vi "OpenNetworkStreamWriter.vi"(6 "E-Stop DVR":refnum<data-value>, 8 "error in (no error)":errorcluster, 11 "Writer Parameters":T1) -> (0 "error out":errorcluster, 2 "Time Opened":timestamp, 3 "Writer Endpoint":refnum<k21>, 4 "Aborted?":bool)   [LabVIEW 2012, in "NetworkStreamWriter.lvclass"]
doc: "Opens a network stream writer endpoint. This VI persistently tries to open the connection until it is successful or the e-stop is triggered by-reference (data value reference). The e-stop will be triggered by the Close method of the owning Object.\n\nJared Kirschner, 2012."
uses:
  NetworkStreamWriter.lvclass
  WriterParameters.ctl
  Shared/ElapsedTimeMessage.ctl
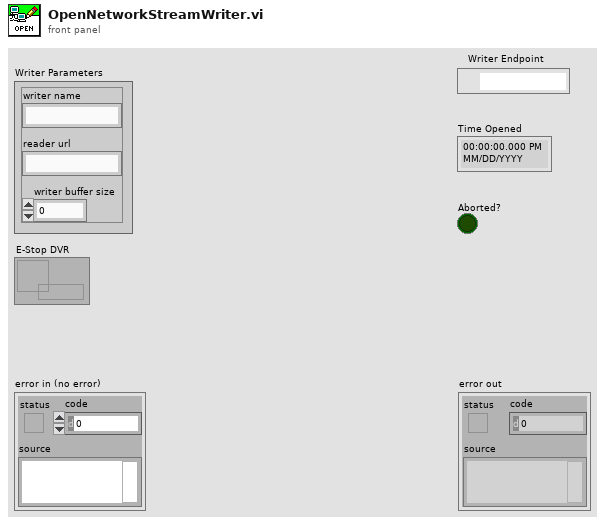
[diagram p1: front panel]
types:
  T1 = typedef "NetworkStreamWriter.lvclass/WriterParameters.ctl" = cluster{"writer name":string, "reader url":string, "writer buffer size":i32}
  T2 = typedef "ElapsedTimeMessage.ctl" = cluster{"Data":variant, "Elapsed Time (s)":dbl}
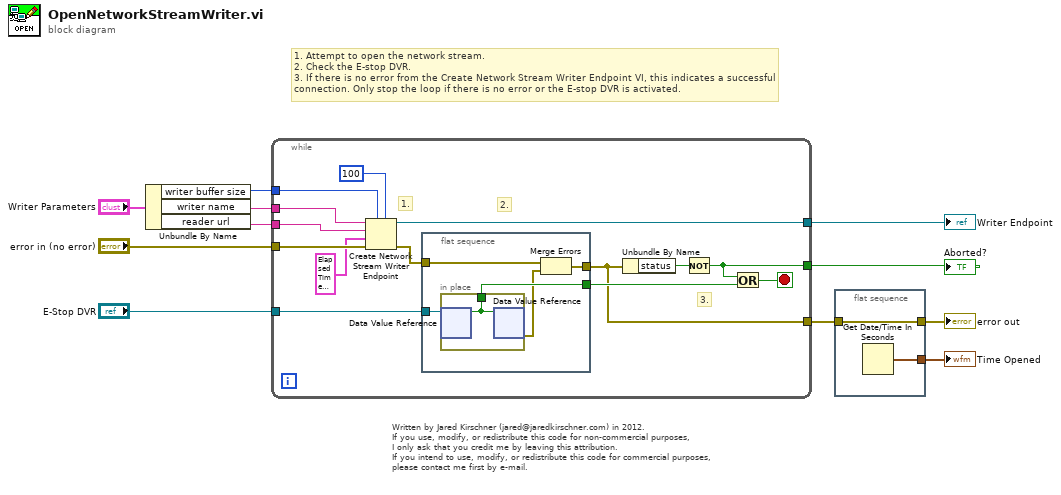
[diagram p0: block diagram]
diagram:
  # "1. Attempt to open the network stream.\n2. Check the E-stop DVR.\n3. If there is no error from the Create Network Stream Writer Endpoint VI, this indicates a successful\nconnection. Only stop the loop if there is no error or the E-stop DVR is activated."
  # "Written by Jared Kirschner (jared@jaredkirschner.com) in 2012.\nIf you use, modify, or redistribute this code for non-commercial purposes,\nI only ask that you credit me by leaving this attribution.\nIf you intend to use, modify, or redistribute this code for commercial purposes,\nplease contact me first by e-mail."
  n1 = Unbundle By Name("Writer Parameters") -> ("writer buffer size"=w8:i32, "writer name"=w7:string, "reader url"=w6:string)
  n2 = while {
    tunnel: "error in (no error)" -> [w25]
    tunnel: w8 -> [w24]
    tunnel: [w12] -> w4
    tunnel: w7 -> [w23]
    tunnel: w6 -> [w22]
    tunnel: [w20] -> w1
    tunnel: [w17] -> w10
    tunnel: "E-Stop DVR" -> [w14]
    stop <- w16 stop-if-true
    # "3."
    # "2."
    # "1."
    n3 = Create Network Stream Writer Endpoint(5:100 ("timeout in ms (-1)"), 7:w24, 8:w25, 9:T2 {"Data"=variant, "Elapsed Time (s)"=0.0} ("variant"), 10:w22, 11:w23) -> (0:w13:errorcluster, 3:w20:refnum<k21>)  [unwired: 1 in]
    n4 = flat-sequence {
      tunnel: [w30] -> w15
      tunnel: w14 -> [w29]
      tunnel: w13 -> [w26]
      tunnel: [w28] -> w12
      frame #0 {
        n5 = in-place {
          in-place-border: [w31] -> w30
          n6 = in-place-dvr #1(w29) -> (w31:bool)  [unwired: 1 out]
          n7 = in-place-dvr #1(w31) -> (w27:errorcluster)  [unwired: 1 out]
        }
        n8 = Merge Errors(w26, w27) -> (w28:errorcluster)
      }
    }
    n9 = Unbundle By Name(w12) -> ("status"=w19:bool)
    n10 = Not(x=w19) -> (.not. x?=w17:bool)
    n11 = Or(x=w17, y=w15) -> (x .or. y?=w16:bool)
  }
  "Aborted?" <- w10
  "Writer Endpoint" <- w1
  n12 = flat-sequence {
    tunnel: w4 -> [w33]
    tunnel: [w33] -> w3
    tunnel: [w32] -> w2
    frame #0 {
      n13 = Get Date/Time In Seconds() -> (seconds since 1Jan1904=w32:timestamp)
    }
  }
  "error out" <- w3
  "Time Opened" <- w2
